vi "Create AMC.vi"(8 "error in (no error)":errorcluster, 10 "message queue name":string, 11 "Model_AMC in":refnum<class "Model_AMC.lvclass">) -> (0 "error out":errorcluster, 3 "Model_AMC out":refnum<class "Model_AMC.lvclass">)   [LabVIEW 2021, in "Model_AMC.lvclass"]
uses:
  Model_AMC.lvclass
  Model_AMC.lvclass/Model_AMC.ctl
  <userlib>/John_Lib/AMC_FW/AMC_FW.lvlib
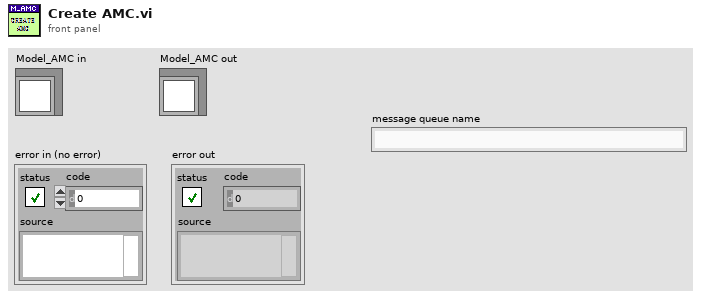
[diagram p1: front panel]
types:
  T1 = typedef "AMC_FW.lvlib/Queue.ctl" = cluster{"Q":T2, "Name":string}
  T2 = typedef "AMC_FW.lvlib/Message Queue.ctl" = refnum<queue>
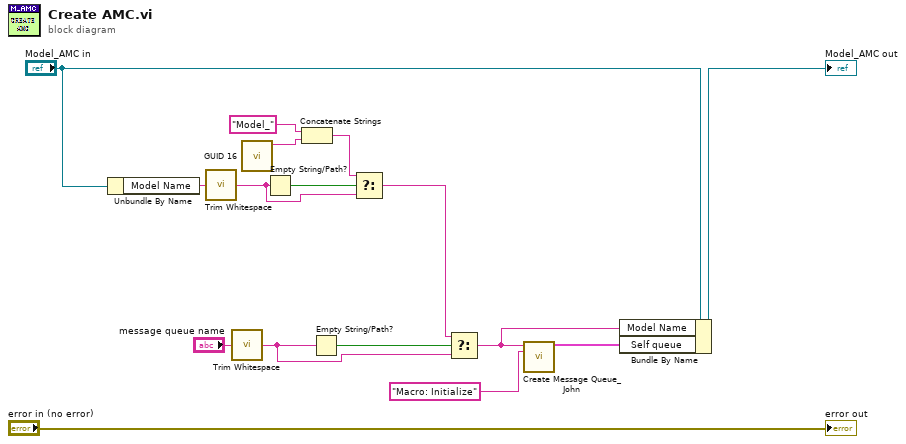
[diagram p0: block diagram]
diagram:
  n1 = Unbundle By Name("Model_AMC in") -> ("Model Name"=w10:string)
  n2 = call <vilib>:"Trim Whitespace.vi"("string"=w10) -> ("trimmed string"=w3:string)  [unwired: 1 in]
  n3 = call <vilib>:"Trim Whitespace.vi"("string"="message queue name") -> ("trimmed string"=w8:string)  [unwired: 1 in]
  n4 = call <userlib>:"GUID 16.vi"() -> ("Hash"=w5:string)  [unwired: 10 in, 1 out]
  n5 = Empty String/Path?(string/path=w3) -> (empty?=w7:bool)
  n6 = Concatenate Strings("Model_" ("message queue name"), w5) -> (w4:string)
  n7 = Empty String/Path?(string/path=w8) -> (empty?=w11:bool)
  n8 = Select(t=w4, s=w7, f=w3) -> (s? t:f=w2:string)
  n9 = Select(t=w2, s=w11, f=w8) -> (s? t:f=w1:string)
  n10 = call <userlib>:"Create Message Queue_John.vi"("message queue name"=w1, "initial message names"="Macro: Initialize") -> ("message queue out"=w13:T1)  [unwired: 12 in, 1 out]
  n11 = Bundle By Name(cluster="Model_AMC in", "Model Name"=w1, "Self queue"=w13) -> (→"Model_AMC out":refnum<class "Model_AMC.lvclass">)
  "error out" <- "error in (no error)"
